vi "PPAS_Command_Globals.vi"() -> ()   [LabVIEW 2019]
panel:
  out "Jim3_Rcvd":bool
  out "Jim2_Rcvd":bool
  out "Jim1_Rcvd":bool
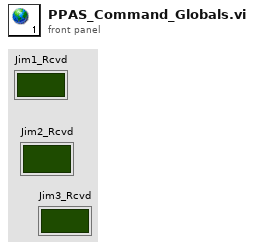
[diagram p1: front panel]
diagram:
